vi "gamepad.vi"   [LabVIEW 2015]
uses:
  <vilib>/LVH/AR Drone Toolkit/AR Drone.lvlib
types:
  T1 = cluster{"Drone IP address":string, "Home IP address":string, "Flight Mode":enum8{"OUTDOOR MODE", "INDOOR MODE"}, "Mounted Hull":enum8{"OUTDOOR HULL", "INDOOR HULL"}, "Video Camera":u8, "Max Altitude (m)":sgl, "Max Pitch and Roll Angle (deg)":sgl, "Max Vertical Speed (m/s)":sgl, "Max Yaw Speed (deg/s)":sgl}
  T2 = cluster{"button 1":bool, "button 2":bool, "button 3":bool, "button 4":bool, "button 5":bool, "button 6":bool, "button 7":bool, "button 8":bool, "button 9":bool, "button 10":bool, "button 11":bool, "button 12":bool, "button 13":bool, "button 14":bool, "button 15":bool, "button 16":bool, "button 17":bool, "button 18":bool, "button 19":bool, "button 20":bool, "button 21":bool, "button 22":bool, "button 23":bool, "button 24":bool, "button 25":bool, "button 26":bool, "button 27":bool, "button 28":bool, "button 29":bool, "button 30":bool, "button 31":bool, "button 32":bool}
  T3 = typedef "AR Drone.lvlib/AR Drone Resource.ctl" = cluster{"UDP Control Connection":refnum<k16>, "UDP NavData Connection":refnum<k16>, "UDP Video Connection (Drone 1.0)":refnum<k16>, "TCP Video Connection (Drone 2.0)":refnum<k5>, "TCP Control Port Connection":refnum<k5>, "Drone IP address":string, "Drone Command Port":u16, "Drone NavData Port":u16, "Drone Vid Stream Port":u16, "Drone TCP Control Port":u16, "Home IP address":string, "Home Command Port":u16, "Home NavData Port":u16, "Home Vid Stream Port":u16, "Drone Version":i32, "Drone Index":i32, "Command Sequence":i32}
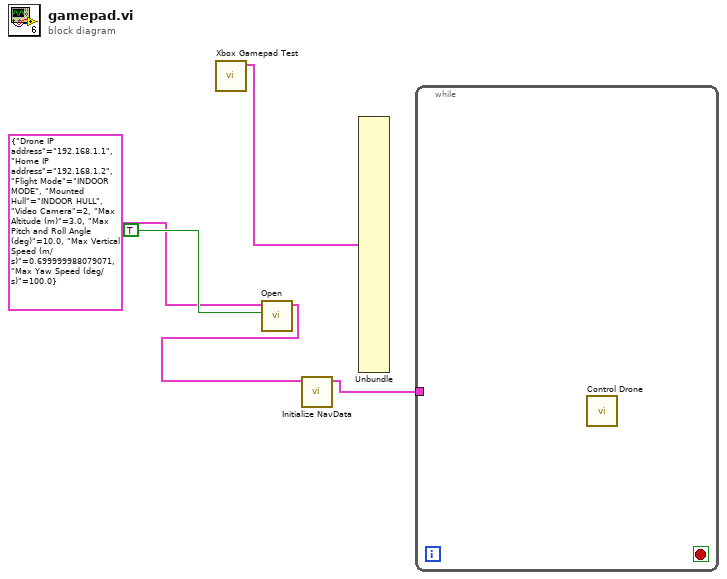
[diagram p0: block diagram]
diagram:
  n1 = call <vilib>:"Xbox Gamepad Test.vi"() -> ("button info"=w1:T2)  [unwired: 10 in, 1 out]
  n2 = call <vilib>:"Open.vi"("Init NavData?"=TRUE, "Setup Parameters"=T1 {"Drone IP address"="192.168.1.1", "Home IP address"="192.168.1.2", "Flight Mode"=enum."INDOOR MODE", "Mounted Hull"=enum."INDOOR HULL", "Video Camera"=2, "Max Altitude (m)"=3.0, "Max Pitch and Roll Angle (deg)"=10.0, "Max Vertical Speed (m/s)"=0.7, "Max Yaw Speed (deg/s)"=100.0}) -> ("AR Drone Resource"=w3:T3)  [unwired: 8 in, 1 out]
  n3 = call <vilib>:"Initialize NavData.vi"("AR Drone Resource"=w3) -> ("AR Drone Resource Out"=w2:T3)  [unwired: 9 in, 1 out]
  n4 = Unbundle(w1) -> ()  [unwired: 32 out]
  n5 = while {
    tunnel: w2 -> [_]
    stop <- _ stop-if-true
    n6 = call <vilib>:"Control Drone.vi"() -> ()  [unwired: 10 in, 2 out]
  }
